vi "Get Sender.vi"(11 "Override Error Msg Strategy in":refnum<class "Override Error Msg Strategy.lvclass">) -> (2 "Sender":refnum<class "Sender.lvclass">)   [LabVIEW 2021, in "Override Error Msg Strategy.lvlib" / "Override Error Msg Strategy.lvclass"]
uses:
  Override Error Msg Strategy.lvclass
  Override Error Msg Strategy.lvclass/Override Error Msg Strategy.ctl
  jettl/Sender/Sender/Sender.lvclass
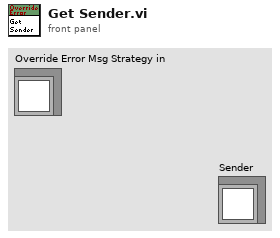
[diagram p1: front panel]
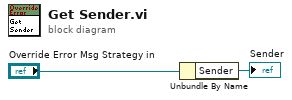
[diagram p0: block diagram]
diagram:
  n1 = Unbundle By Name("Override Error Msg Strategy in") -> ("Sender"=→"Sender":refnum<class "Sender.lvclass">)
